vi "Log Message - CRITICAL.vi"(6 "error in (no error)":errorcluster, 7 "Message":string) -> (2 "error out":errorcluster)   [LabVIEW 2020, in "RxnRover.lvlib" / "logging.lvlib"]
doc: "Log the given message to the Rxn Rover log file with log level CRITICAL."
uses:
  logging.lvlib
  Levels.ctl
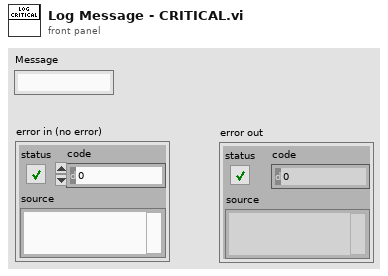
[diagram p1: front panel]
types:
  T1 = typedef "RxnRover.lvlib/logging.lvlib/Levels.ctl" = enum16{"NOTSET", "DEBUG", "INFO", "WARNING", "ERROR", "CRITICAL"}
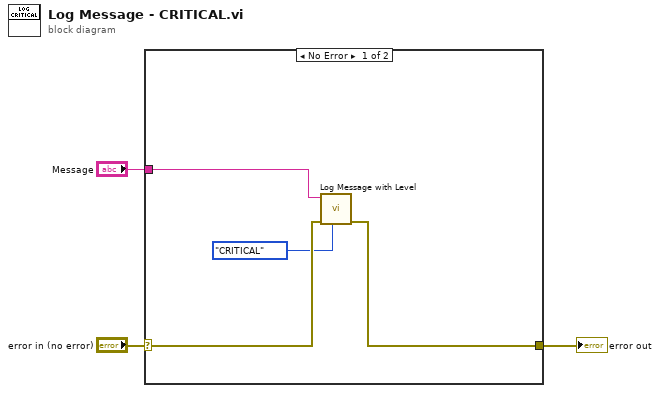
[diagram p0: block diagram]
diagram:
  n1 = case shown="No Error" "error in (no error)" {
    selector: "error in (no error)" -> [w6 w8]
    tunnel: [w7 w8] -> w2
    tunnel: "Message" -> [w5 _]
    frame No Error {
      n2 = call "Log Message with Level.vi"("Log Level (INFO)"=Levels."CRITICAL", "error in (no error)"=w6, "Message"=w5) -> ("error out"=w7:errorcluster)  [unwired: 8 in]
    }
    frame Error {
    }
  }
  "error out" <- w2
